vi "grab_qrcode_nivision.vi"() -> ()   [LabVIEW 2018]
uses:
  <vilib>/userdefined/High Color/IMAQdx.ctl
  <vilib>/vision/driver/NI_Vision_Acquisition_Software.lvlib
  <vilib>/vision/NI_Vision_Development_Module.lvlib
panel:
  out "Image":T1(plugin-control)
  in  "stop":bool
  out "return value":cluster{"found":i32, "decode data":string}
  in  "Output image filename":string="decode.png"
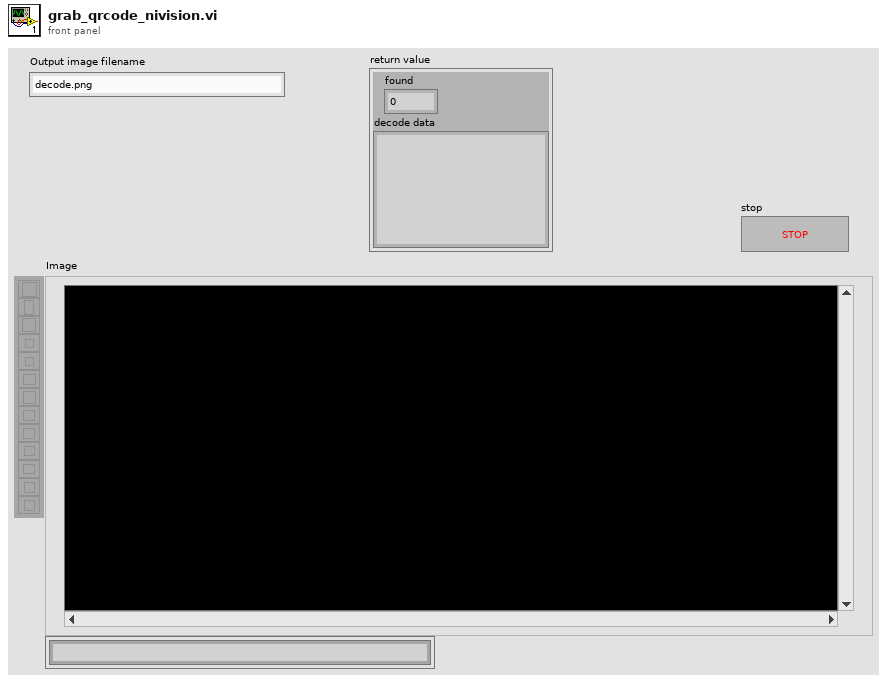
[diagram p1: front panel]
types:
  T1 = typedef "IMAQ Image.ctl" = refnum<image>
  T2 = typedef "Image Type" = u32
  T3 = typedef "IMAQdx.ctl" = refnum<k21>
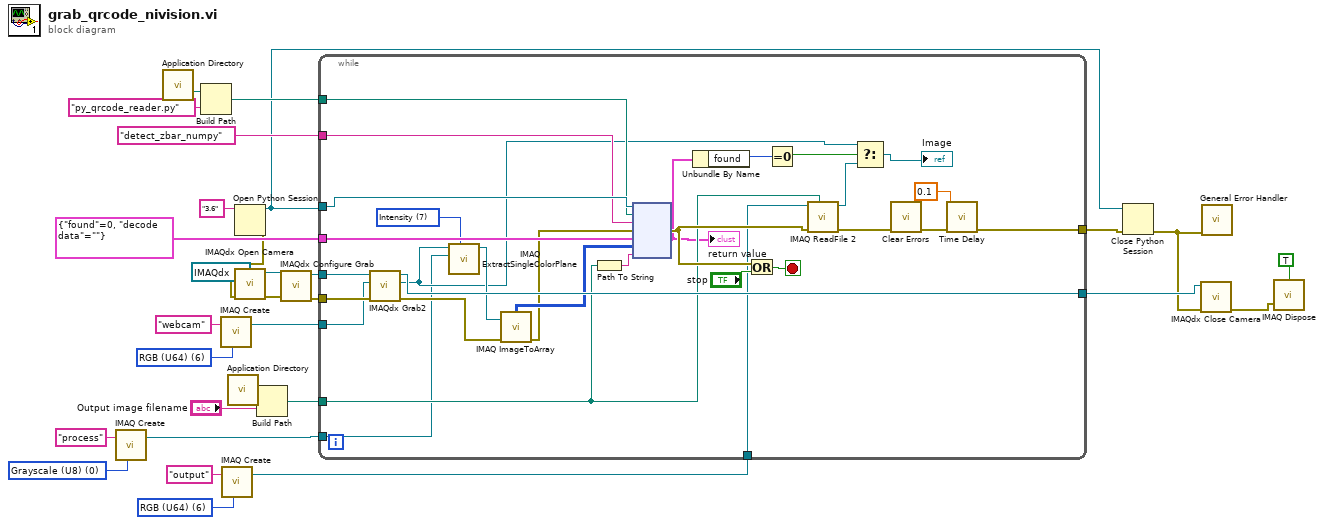
[diagram p0: block diagram]
diagram:
  w4 = T2 0 items=["Grayscale (U8)", "Grayscale (I16)", "Grayscale (SGL)", "Complex (CSG)", "RGB (U32)", "HSL (U32)", "RGB (U64)", "Grayscale (U16)"] ("Image Type")
  w7 = T2 6 items=["Grayscale (U8)", "Grayscale (I16)", "Grayscale (SGL)", "Complex (CSG)", "RGB (U32)", "HSL (U32)", "RGB (U64)", "Grayscale (U16)"] ("Image Type")
  w9 = T2 6 items=["Grayscale (U8)", "Grayscale (I16)", "Grayscale (SGL)", "Complex (CSG)", "RGB (U32)", "HSL (U32)", "RGB (U64)", "Grayscale (U16)"] ("Image Type")
  n1 = call "IMAQ Create"("Image Name"="process", "Image Type"=w4) -> ("New Image"=w3:T1)  [unwired: 3 in, 1 out]
  n2 = call <vilib>:"Application Directory.vi"() -> ("Application Directory"=w28:path)
  n3 = Build Path(base path=w28, name or relative path="py_qrcode_reader.py" ("module filename")) -> (appended path=w26:path)
  n4 = call "IMAQ Create"("Image Name"="webcam", "Image Type"=w9) -> ("New Image"=w10:T1)  [unwired: 3 in, 1 out]
  n5 = call "IMAQ Create"("Image Name"="output", "Image Type"=w7) -> ("New Image"=w6:T1)  [unwired: 3 in, 1 out]
  n6 = call <vilib>:"Application Directory.vi"() -> ("Application Directory"=w22:path)
  n7 = Open Python Session(python version="3.6" ("Python version")) -> (session out=w24:refnum<k35>, error out=w13:errorcluster)  [unwired: 2 in]
  n8 = call <vilib>:"IMAQdx Open Camera.vi"("error in"=w13, "Session In"=T3 "cam0") -> ("error out"=w19:errorcluster, "Session Out"=w18:T3)  [unwired: 8 in]
  n9 = Build Path(base path=w22, name or relative path="Output image filename") -> (appended path=w20:path)
  n10 = call <vilib>:"IMAQdx Configure Grab.vi"("error in"=w19, "Session In"=w18) -> ("error out"=w16:errorcluster, "Session Out"=w17:T3)  [unwired: 8 in]
  n11 = while {
    tunnel: w24 -> [w60]
    tunnel: "detect_zbar_numpy" ("function name") -> [w59]
    tunnel: cluster{"found":i32, "decode data":string} {"found"=0, "decode data"=""} -> [w58]
    tunnel: w26 -> [w57]
    tunnel: [w52] -> w25
    tunnel: w20 -> [w40]
    tunnel: w17 -> [w51]
    tunnel: w16 -> [w50]
    tunnel: [w49] -> w15
    tunnel: w10 -> [w31]
    tunnel: w6 -> [w41]
    tunnel: w3 -> [w32]
    stop <- w55 stop-if-true
    w45 = 7 items=["Red", "Green", "Blue", "Hue", "Saturation", "Luminance", "Value", "Intensity"] ("Color Plane")
    n12 = call <vilib>:"IMAQdx Grab2.vi"("error in"=w50, "Image In"=w31, "Session In"=w51) -> ("error out"=w47:errorcluster, "Image Out"=w33:T1, "Session Out"=w49:T3)  [unwired: 5 in, 1 out]
    n13 = call "IMAQ ExtractSingleColorPlane"("Color Plane"=w45, "Image Dst"=w32, "Image Src"=w33) -> ("Image Dst Out"=w44:T1)  [unwired: 7 in, 1 out]
    n14 = call "IMAQ ImageToArray"("error in (no error)"=w47, "Image"=w44) -> ("error out"=w46:errorcluster, "Image Pixels (U8)"=w48:u8[][])  [unwired: 2 in, 3 out]
    n15 = Path To String(path=w40) -> (string=w53:string)
    n16 = node(w60, w57, w59, w46, w58, w48, w53) -> (w42:errorcluster, w38:cluster{"found":i32, "decode data":string})  [unwired: 2 in, 3 out]
    "return value" <- w38
    n17 = Unbundle By Name(w38) -> ("found"=w37:i32)
    n18 = Or(x=w42, y="stop") -> (x .or. y?=w55:bool)
    n19 = Equal To 0?(x=w37) -> (x = 0?=w36:bool)
    n20 = call "IMAQ ReadFile 2"("File Path"=w40, "error in (no error)"=w42, "Image"=w41) -> ("error out"=w39:errorcluster, "Image Out"=w35:T1)  [unwired: 4 in, 3 out]
    n21 = Select(t=w33, s=w36, f=w35) -> (s? t:f=→"Image":T1)
    n22 = call <vilib>:"Clear Errors.vi"("error in (no error)"=w39) -> ("error out"=w54:errorcluster)  [unwired: 5 in, 1 out]
    n23 = call "Time Delay"("error in (no error)"=w54, "Delay Time (s)"=0.1) -> ("error out"=w52:errorcluster)  [unwired: 9 in]
  }
  n24 = Close Python Session(session in=w24, error in=w25) -> (11:w14:errorcluster)
  n25 = call <vilib>:"IMAQdx Close Camera.vi"("error in"=w14, "Session In"=w15) -> ("error out"=w2:errorcluster)  [unwired: 9 in]
  n26 = call <vilib>:"General Error Handler.vi"("error in (no error)"=w14) -> ()  [unwired: 10 in, 5 out]
  n27 = call "IMAQ Dispose"("All Images? (No)"=TRUE, "error in (no error)"=w2) -> ()  [unwired: 4 in, 1 out]
